vi "produce last data.vi"(11 "Array":string[][](array[string])) -> (1 "Numeric 4":dbl, 2 "Numeric 5":dbl, 3 "Numeric 6":dbl, 4 "Numeric 3":dbl, 5 "Numeric":dbl, 6 "Numeric 2":dbl)   [LabVIEW 2018]
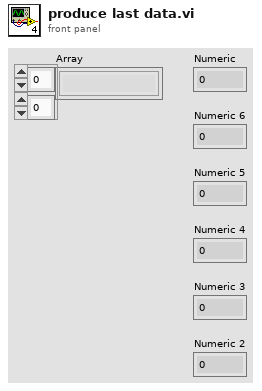
[diagram p1: front panel]
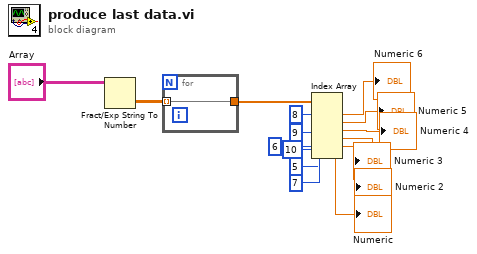
[diagram p0: block diagram]
diagram:
  n1 = Fract/Exp String To Number(string="Array") -> (number=w1:dbl[][])  [unwired: 3 in, 1 out]
  n2 = for {
    tunnel: w1 -> [w16] mode=indexing
    tunnel: [w16] -> w3
  }
  n3 = Index Array(array=w3, index #1=8 ("index"), index #2=9 ("index"), index #3=10 ("index"), index #4=5 ("index"), index #5=6 ("index"), index #6=7 ("index")) -> (element #1=→"Numeric 6":dbl, element #2=→"Numeric 5":dbl, element #3=→"Numeric 4":dbl, element #4=→"Numeric 3":dbl, element #5=→"Numeric 2":dbl, element #6=→"Numeric":dbl)
